vi "RTDE.vi"() -> ()   [LabVIEW 2021]
uses:
  Z:/Samples/LabVIEW/Library/UnderAutomation.UniversalRobots.dll
  Library/UnderAutomation.UniversalRobots.dll
panel:
  out "Connected":bool
  out "Error logs":string
  out "Connect error":errorcluster
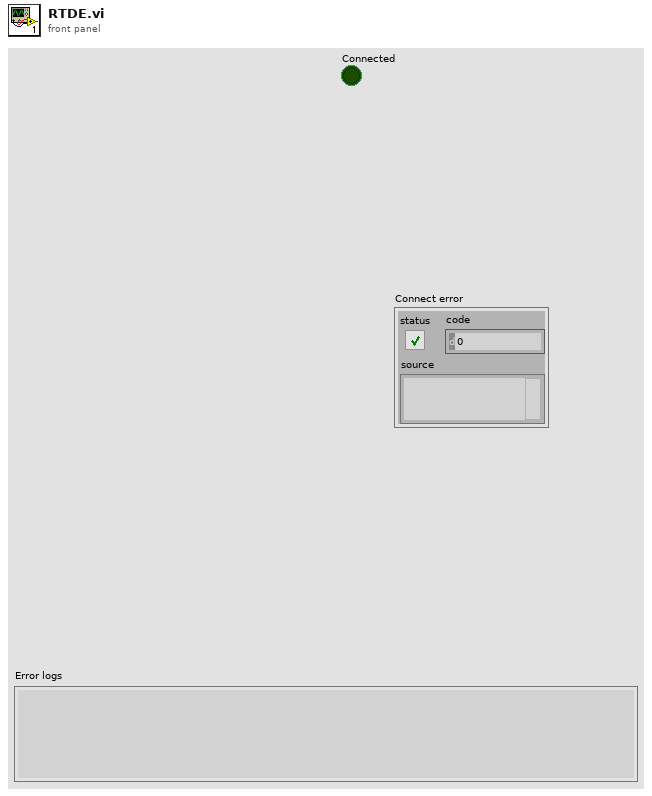
[diagram p1: front panel]
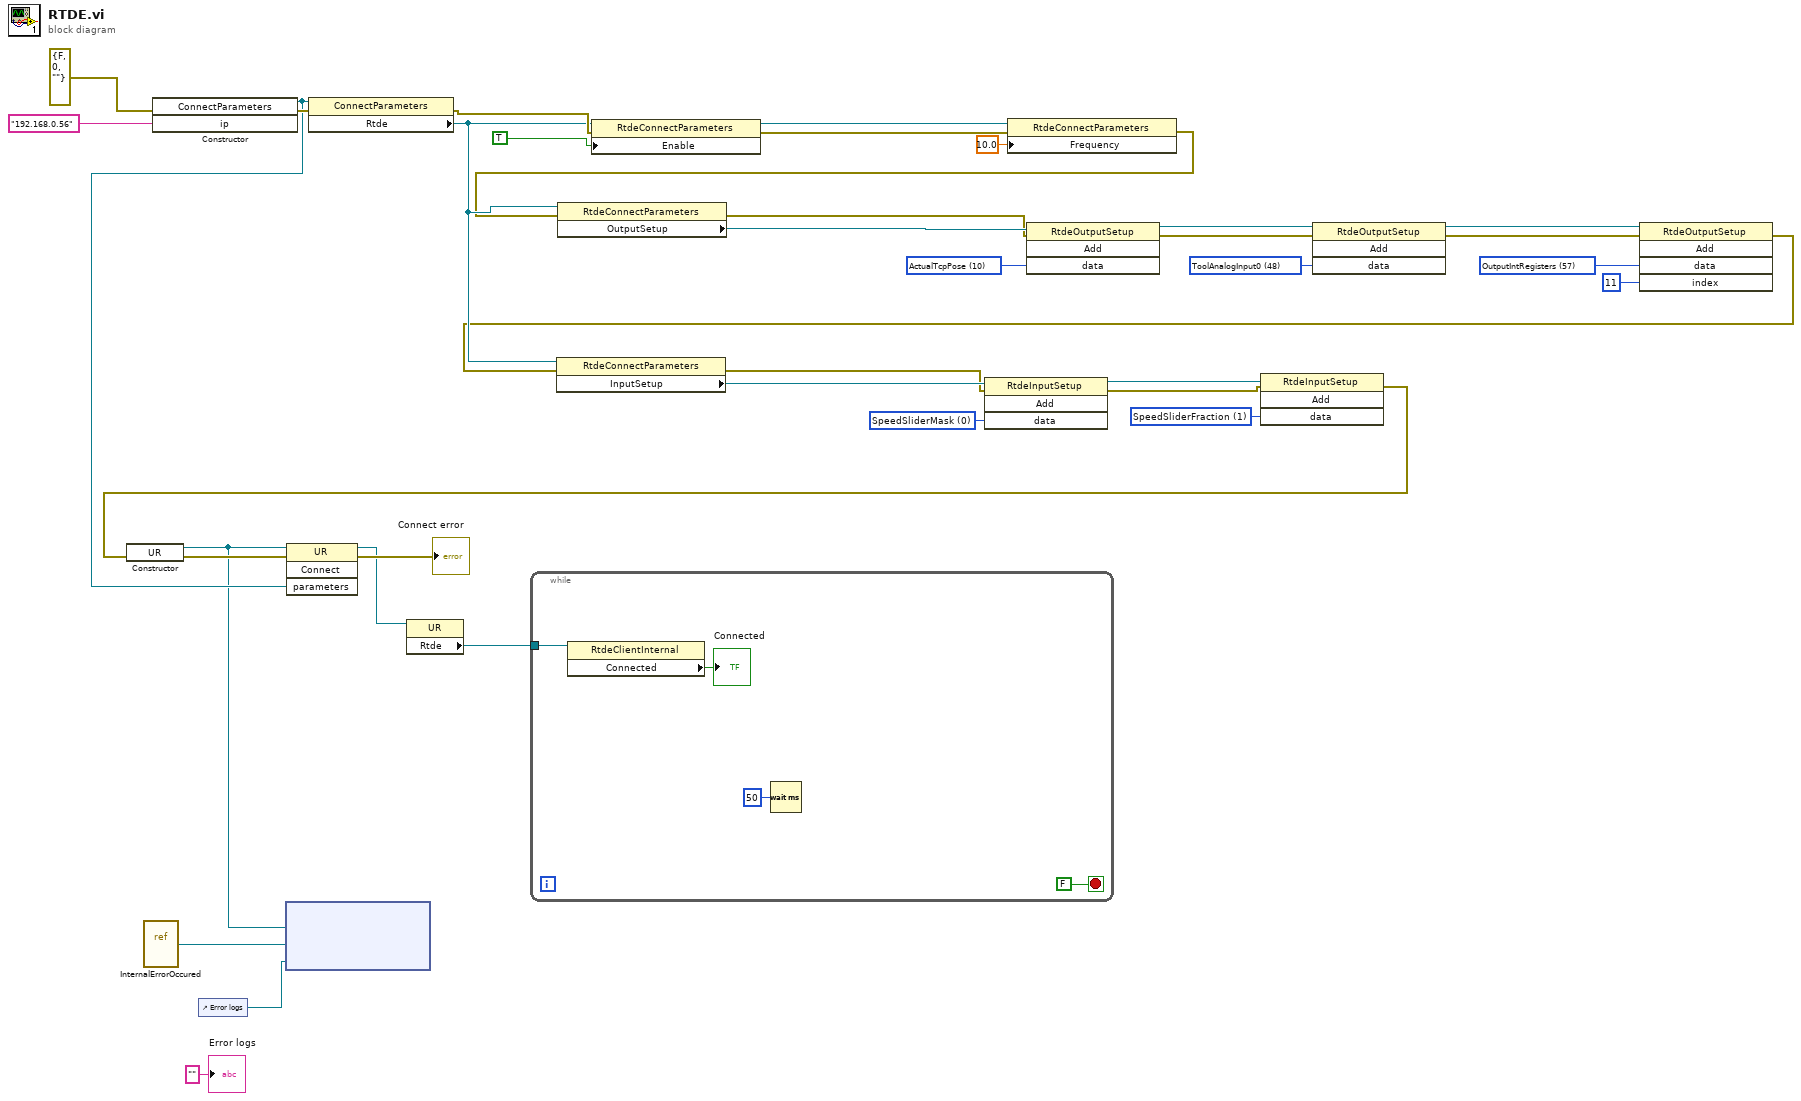
[diagram p0: block diagram]
diagram:
  w19 = 1 items=["SpeedSliderMask", "SpeedSliderFraction", "StandardDigitalOutputMask", "ConfigurableDigitalOutputMask", "StandardDigitalOutput", "ConfigurableDigitalOutput", "StandardAnalogOutputMask", "StandardAnalogOutputType", "StandardAnalogOutput0", "StandardAnalogOutput1", "InputBtRegisters0To31", "InputBtRegisters32To63", "InputBitRegisters", "InputIntRegisters", "InputDoubleRegisters", "ExternalForceTorque"] ("data")
  w21 = 0 items=["SpeedSliderMask", "SpeedSliderFraction", "StandardDigitalOutputMask", "ConfigurableDigitalOutputMask", "StandardDigitalOutput", "ConfigurableDigitalOutput", "StandardAnalogOutputMask", "StandardAnalogOutputType", "StandardAnalogOutput0", "StandardAnalogOutput1", "InputBtRegisters0To31", "InputBtRegisters32To63", "InputBitRegisters", "InputIntRegisters", "InputDoubleRegisters", "ExternalForceTorque"] ("data")
  w31 = 57 items=["Timestamp", "TargetQ", "TargetQd", "TargetQdd", "TargetCurrent", "TargetMoment", "ActualQ", "ActualQd", "ActualCurrent", "JointControlOutput", "ActualTcpPose", "ActualTcpSpeed", "ActualTcpForce", "TargetTcpPose", "TargetTcpSpeed", "ActualDigitalInputBits", "JointTemperatures", "ActualExecutionTime", "RobotMode", "JointMode", "SafetyMode", "SafetyStatus", "ActualToolAccelerometer", "SpeedScaling", "TargetSpeedFraction", "ActualMomentum", "ActualMainVoltage", "ActualRobotVoltage", "ActualRobotCurrent", "ActualJointVoltage", "ActualDigitalOutputBits", "RuntimeState", "ElbowPosition", "ElbowVelocity", "RobotStatusBits", "SafetyStatusBits", "AnalogIOTypes", "StandardAnalogInput0", "StandardAnalogInput1", "StandardAnalogOutput0", "StandardAnalogOutput1", "IOCurrent", "Euromap67InputBits", "Euromap67OutputBits", "Euromap67_24VVoltage", "Euromap67_24VCurrent", "ToolMode", "ToolAnalogInputTypes", "ToolAnalogInput0", "ToolAnalogInput1", "ToolOutputVoltage", "ToolOutputCurrent", "ToolTemperature", "TcpForceScalar", "OutputBitRegisters0To31", "OutputBitRegisters32To63", "OutputBitRegisters", "OutputIntRegisters", "OutputDoubleRegisters", "InputBitRegisters0To31", "InputBitRegisters32To63", "InputBitRegisters", "InputIntRegisters", "InputDoubleRegisters", "ToolOutputMode", "ToolDigitalOutput0mode", "ToolDigitalOutput1Mode", "Payload", "PayloadCOG", "PayloadInertia", "ScriptControlLine", "FTRawWrench"] ("data")
  w33 = 48 items=["Timestamp", "TargetQ", "TargetQd", "TargetQdd", "TargetCurrent", "TargetMoment", "ActualQ", "ActualQd", "ActualCurrent", "JointControlOutput", "ActualTcpPose", "ActualTcpSpeed", "ActualTcpForce", "TargetTcpPose", "TargetTcpSpeed", "ActualDigitalInputBits", "JointTemperatures", "ActualExecutionTime", "RobotMode", "JointMode", "SafetyMode", "SafetyStatus", "ActualToolAccelerometer", "SpeedScaling", "TargetSpeedFraction", "ActualMomentum", "ActualMainVoltage", "ActualRobotVoltage", "ActualRobotCurrent", "ActualJointVoltage", "ActualDigitalOutputBits", "RuntimeState", "ElbowPosition", "ElbowVelocity", "RobotStatusBits", "SafetyStatusBits", "AnalogIOTypes", "StandardAnalogInput0", "StandardAnalogInput1", "StandardAnalogOutput0", "StandardAnalogOutput1", "IOCurrent", "Euromap67InputBits", "Euromap67OutputBits", "Euromap67_24VVoltage", "Euromap67_24VCurrent", "ToolMode", "ToolAnalogInputTypes", "ToolAnalogInput0", "ToolAnalogInput1", "ToolOutputVoltage", "ToolOutputCurrent", "ToolTemperature", "TcpForceScalar", "OutputBitRegisters0To31", "OutputBitRegisters32To63", "OutputBitRegisters", "OutputIntRegisters", "OutputDoubleRegisters", "InputBitRegisters0To31", "InputBitRegisters32To63", "InputBitRegisters", "InputIntRegisters", "InputDoubleRegisters", "ToolOutputMode", "ToolDigitalOutput0mode", "ToolDigitalOutput1Mode", "Payload", "PayloadCOG", "PayloadInertia", "ScriptControlLine", "FTRawWrench"] ("data")
  w35 = 10 items=["Timestamp", "TargetQ", "TargetQd", "TargetQdd", "TargetCurrent", "TargetMoment", "ActualQ", "ActualQd", "ActualCurrent", "JointControlOutput", "ActualTcpPose", "ActualTcpSpeed", "ActualTcpForce", "TargetTcpPose", "TargetTcpSpeed", "ActualDigitalInputBits", "JointTemperatures", "ActualExecutionTime", "RobotMode", "JointMode", "SafetyMode", "SafetyStatus", "ActualToolAccelerometer", "SpeedScaling", "TargetSpeedFraction", "ActualMomentum", "ActualMainVoltage", "ActualRobotVoltage", "ActualRobotCurrent", "ActualJointVoltage", "ActualDigitalOutputBits", "RuntimeState", "ElbowPosition", "ElbowVelocity", "RobotStatusBits", "SafetyStatusBits", "AnalogIOTypes", "StandardAnalogInput0", "StandardAnalogInput1", "StandardAnalogOutput0", "StandardAnalogOutput1", "IOCurrent", "Euromap67InputBits", "Euromap67OutputBits", "Euromap67_24VVoltage", "Euromap67_24VCurrent", "ToolMode", "ToolAnalogInputTypes", "ToolAnalogInput0", "ToolAnalogInput1", "ToolOutputVoltage", "ToolOutputCurrent", "ToolTemperature", "TcpForceScalar", "OutputBitRegisters0To31", "OutputBitRegisters32To63", "OutputBitRegisters", "OutputIntRegisters", "OutputDoubleRegisters", "InputBitRegisters0To31", "InputBitRegisters32To63", "InputBitRegisters", "InputIntRegisters", "InputDoubleRegisters", "ToolOutputMode", "ToolDigitalOutput0mode", "ToolDigitalOutput1Mode", "Payload", "PayloadCOG", "PayloadInertia", "ScriptControlLine", "FTRawWrench"] ("data")
  n1 = vi-ref "InternalErrorOccured.vi"() -> ("vi reference"=w2:refnum<vi>)
  n2 = constructor class="ConnectParameters"(error in=errorcluster {"status"=FALSE, "code"=0, "source"=""} ("error in (no error)"), "ip"="192.168.0.56") -> (reference out=w9:refnum<k24>, error out=w28:errorcluster)  [unwired: 2 in, 2 out]
  n3 = control-ref of="Error logs"() -> (w3:refnum<vi>)
  n4 = property class="ConnectParameters"(reference=w9, error in=w28) -> (error out=w27:errorcluster, "Rtde"=w23:refnum<k24>)  [unwired: 1 out]
  n5 = property class="RtdeConnectParameters"(reference=w23, error in=w27, "Enable"=TRUE) -> (reference out=w15:refnum<k24>, error out=w13:errorcluster)
  n6 = property class="RtdeConnectParameters"(reference=w15, error in=w13, "Frequency"=10.0) -> (error out=w12:errorcluster)  [unwired: 1 out]
  n7 = property class="RtdeConnectParameters"(reference=w23, error in=w12) -> (error out=w26:errorcluster, "OutputSetup"=w36:refnum<k24>)  [unwired: 1 out]
  n8 = invoke class="RtdeOutputSetup" method="Add"(reference=w36, error in=w26, "data"=w35) -> (reference out=w34:refnum<k24>, error out=w25:errorcluster)  [unwired: 1 in, 2 out]
  n9 = invoke class="RtdeOutputSetup" method="Add"(reference=w34, error in=w25, "data"=w33) -> (reference out=w32:refnum<k24>, error out=w24:errorcluster)  [unwired: 1 in, 2 out]
  n10 = invoke class="RtdeOutputSetup" method="Add"(reference=w32, error in=w24, "data"=w31, "index"=11) -> (error out=w18:errorcluster)  [unwired: 1 in, 4 out]
  n11 = property class="RtdeConnectParameters"(reference=w23, error in=w18) -> (error out=w17:errorcluster, "InputSetup"=w22:refnum<k24>)  [unwired: 1 out]
  n12 = invoke class="RtdeInputSetup" method="Add"(reference=w22, error in=w17, "data"=w21) -> (reference out=w20:refnum<k24>, error out=w16:errorcluster)  [unwired: 1 in, 2 out]
  n13 = invoke class="RtdeInputSetup" method="Add"(reference=w20, error in=w16, "data"=w19) -> (error out=w10:errorcluster)  [unwired: 1 in, 3 out]
  n14 = constructor class="UR"(error in=w10) -> (reference out=w4:refnum<k24>, error out=w11:errorcluster)  [unwired: 2 in, 1 out]
  n15 = node(w4, w2, w3) -> ()  [unwired: 2 in, 2 out]
  n16 = invoke class="UR" method="Connect"(reference=w4, error in=w11, "parameters"=w9) -> (reference out=w6:refnum<k24>, error out=→"Connect error":errorcluster)  [unwired: 1 in, 2 out]
  n17 = property class="UR"(reference=w6) -> ("Rtde"=w5:refnum<k24>)  [unwired: 1 in, 2 out]
  n18 = while {
    tunnel: w5 -> [w41]
    stop <- FALSE stop-if-true
    n19 = property class="RtdeClientInternal"(reference=w41) -> ("Connected"=→"Connected":bool)  [unwired: 1 in, 2 out]
    n20 = Wait (ms)(milliseconds to wait=u32 50) -> ()  [unwired: 1 out]
  }
  "Error logs" <- "" ("Error logs")
